vi "Set Z Piezo_test.vi"(4 "X Offset Voltage":dbl caption="Offset" min=-10.0 max=10.0 step=0.1) -> ()   [LabVIEW 2014]
uses:
  Instance           1 19Saved   Set Stage Z .vi
  Instance           2 19Saved   Set Stage Z .vi
panel:
  in  "Case Constant\n(See Context Help)":bool
  out "Numeric":dbl
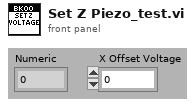
[diagram p1: front panel]
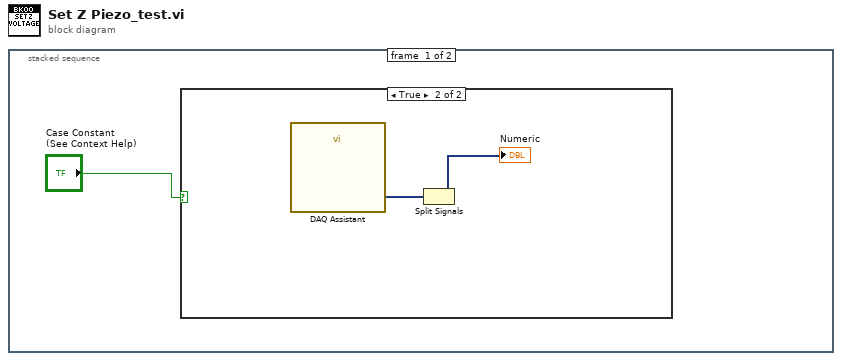
[diagram p0: block diagram]
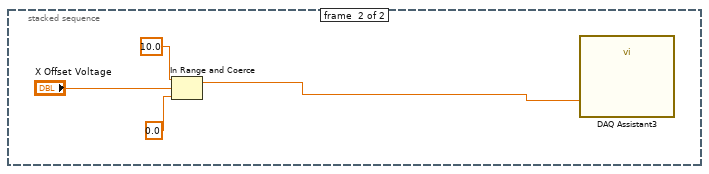
[diagram p3: hidden frame]
diagram:
  n1 = stacked-sequence {
    frame #0 {
      n2 = case shown="True" "Case Constant\n(See Context Help)" {
        frame False {
        }
        frame True {
          n3 = call "DAQ Assistant"() -> ("data"=w2:dynamicdata)  [unwired: 17 in, 2 out]
          n4 = Split Signals(w2) -> (→"Numeric":dynamicdata)  [unwired: 2 in, 1 out]
        }
      }
    }
    frame #1 {
      n5 = In Range and Coerce(upper limit=10.0, x="X Offset Voltage", lower limit=0.0) -> (coerced(x)=w4:dbl)  [unwired: 1 out]
      n6 = call "DAQ Assistant3"("data"=w4) -> ()  [unwired: 17 in, 2 out]
    }
  }
